vi "Release.vi"(8 "error in (no error)":errorcluster, 11 "CallRequest (JSON) in":refnum<class "CallRequest (JSON).lvclass">) -> (0 "error out":errorcluster)   [LabVIEW 2020, in "wamplv.lvlib" / "CallRequest (JSON).lvclass"]
uses:
  CallRequest (JSON).lvclass
  CallRequest (JSON).lvclass/CallRequest (JSON).ctl
  4e4b81f5-c4b8-4ae4-8d81-c83602a4892b.vi
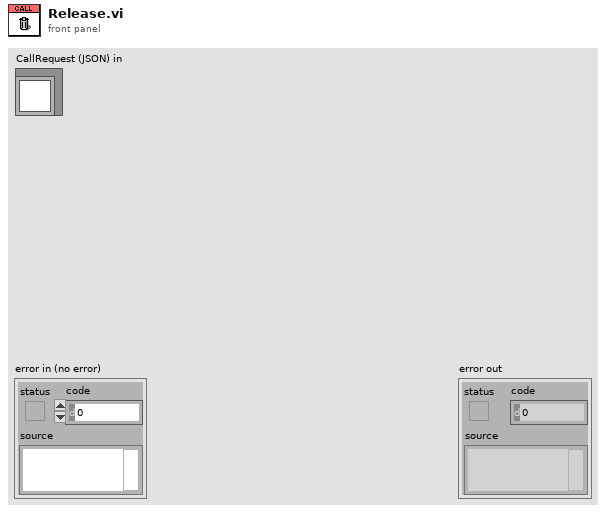
[diagram p1: front panel]
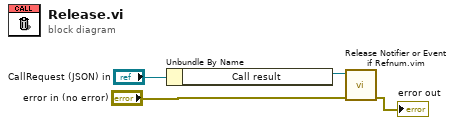
[diagram p0: block diagram]
diagram:
  n1 = Unbundle By Name("CallRequest (JSON) in") -> ("Call result"=w3:refnum<notifier>)
  n2 = call "Release Notifier or Event if Refnum.vim"("error in (no error)"="error in (no error)", "Notifier or Event in"=w3) -> ("error out"=→"error out":errorcluster)  [unwired: 9 in]
